vi "Get DAQ Physical Channels.vi"(8 "error in (no error)":errorcluster, 11 "DAQ Channel Section Refs":T1[](array[typedef]) format="%.0x") -> (0 "error out":errorcluster, 3 "Physical Channels":i32[](array[numeric]))   [LabVIEW 2020, in "Waveform Analog Output Engine.lvlib"]
doc: "Gets the array of physical channels that have been added to the custom device by reading the Physical Channel property of each section reference provided"
uses:
  Waveform Analog Output Engine.lvlib
  <vilib>/NI VeriStand/Custom Device API/Custom Device Item Ref.ctl
  Shared/Constants.vi
  <vilib>/NI VeriStand/Custom Device API/Get Item Property (Variant).vi
  <vilib>/NI VeriStand/Custom Device API/Custom Device API.lvlib
  Shared/Waveform Analog Output Shared.lvlib
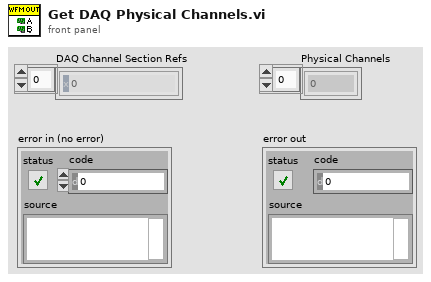
[diagram p1: front panel]
types:
  T1 = typedef "Custom Device API.lvlib/Custom Device Item Ref.ctl" = u64
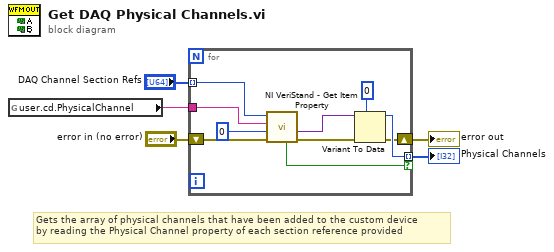
[diagram p0: block diagram]
diagram:
  # "Gets the array of physical channels that have been added to the custom device\nby reading the Physical Channel property of each section reference provided"
  n1 = global read "Constants.vi" "user.cd.PhysicalChannel"() -> (w2:string)
  n2 = for {
    tunnel: "DAQ Channel Section Refs" -> [w15] mode=indexing
    tunnel: w2 -> [w14]
    tunnel: [w9] -> w5 mode=indexing if=w8
    shift-right: [w7] -> w3
    shift-left: "error in (no error)" -> [w6]
    n3 = call-poly <vilib>:"NI VeriStand - Get Item Property.vi"("error in (no error)"=w6, "Default Value"=0, "Property Name"=w14, "Item Ref in"=w15) -> ("error out"=w12:errorcluster, "Value"=w13:variant, "Found?"=w8:bool)  [unwired: 4 in, 1 out]
    n4 = Variant To Data(error in=w12, type=0, Variant=w13) -> (data=w9:i32, error out=w7:errorcluster)
  }
  "Physical Channels" <- w5
  "error out" <- w3
